vi "FT10_Stop Notifier.vi"(7 "Selector":T1, 8 "error in (no error)":errorcluster) -> (0 "error out":errorcluster, 3 "Notifier out":refnum<notifier>)   [LabVIEW 2015]
uses:
  Controls/Config_Stop Notifier Enum.ctl
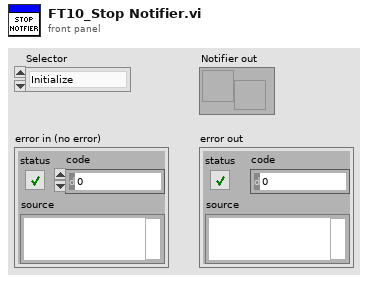
[diagram p1: front panel]
types:
  T1 = typedef "Config_Stop Notifier Enum.ctl" = enum16{"Initialize", "Read Notifier", "Notify", "Close"}
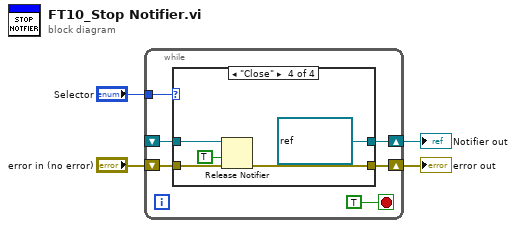
[diagram p0: block diagram]
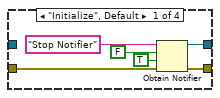
[diagram p2: hidden frame]
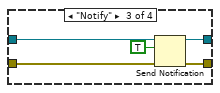
[diagram p4: hidden frame]
diagram:
  n1 = while {
    tunnel: "Selector" -> [w9]
    shift-right: [w6] -> w1
    shift-left: _ -> [w5]
    shift-right: [w7] -> w2
    shift-left: "error in (no error)" -> [w8]
    stop <- TRUE stop-if-true
    n2 = case shown="\"Close\"" w9 {
      tunnel: w8 -> [w13 w17 w23 w27]
      tunnel: [w12 w17 w22 w26] -> w7
      tunnel: [w11 w18 w21 refnum<notifier> refnum ("notifier out")] -> w6
      tunnel: w5 -> [_ w18 w20 w28]
      frame "Initialize", Default {
        n3 = Obtain Notifier(name (unnamed)="Stop Notifier", notification data type=FALSE, create if not found? (T)=TRUE, error in (no error)=w13) -> (notifier out=w11:refnum<notifier>, error out=w12:errorcluster)  [unwired: 1 out]
      }
      frame "Read Notifier" {
      }
      frame "Notify" {
        n4 = Send Notification(notification=TRUE, notifier=w20, error in (no error)=w23) -> (notifier out=w21:refnum<notifier>, error out=w22:errorcluster)
      }
      frame "Close" {
        n5 = Release Notifier(notifier=w28, force destroy? (F)=TRUE, error in (no error)=w27) -> (error out=w26:errorcluster)  [unwired: 2 out]
      }
    }
  }
  "error out" <- w2
  "Notifier out" <- w1
